vi "RTD Read.vi"(0 "Message Queues":T1, 3 "error in":errorcluster) -> (10 "error out":errorcluster)   [LabVIEW 2018, in "RTD.lvlib"]
uses:
  RTD.lvlib
  support/Message Queue/All Message Queues.ctl
  support/Message Queue/Message Cluster.ctl
  TT Configuration.ctl
  <vilib>/DAQmx/read.llb/DAQmx Read (Analog Wfm 1Chan 1Samp).vi
  <vilib>/DAQmx/create/channels.llb/DAQmx Create Channel (AI-Temperature-RTD).vi
  <vilib>/DAQmx/miscellaneous.llb/DAQmx Fill In Error Info.vi
  support/Message Queue/Enqueue Message (Array).vi
  support/Message Queue/Message Queue.lvlib
  Measure Instrument/Feed Module Engine.lvlib
panel:
  in  "TT Configuration":T2={"physical channels"="cDAQ2Mod4/ai0", "name to assign"="Temp1", "units"=10143} {"units" items=["Deg C"=10143, "Deg F"=10144, "Kelvins"=10325, "Deg R"=10145, "From Custom Scale"=10065]}
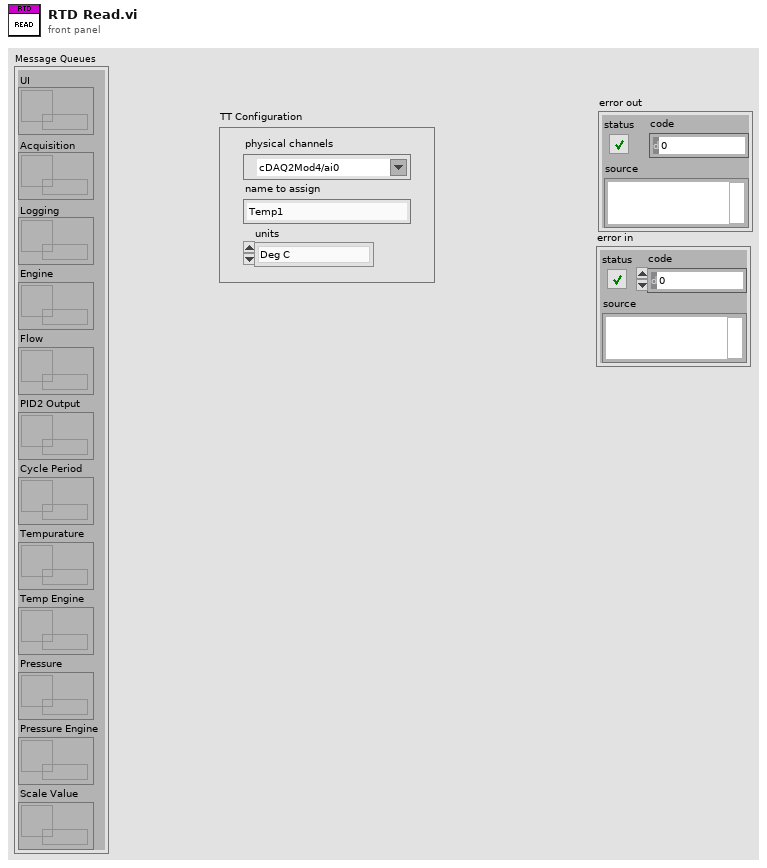
[diagram p1: front panel]
types:
  T1 = typedef "Message Queue.lvlib/All Message Queues.ctl" = cluster{"UI":refnum<queue>, "Acquisition":refnum<queue>, "Logging":refnum<queue>, "Engine":refnum<queue>, "Flow":refnum<queue>, "PID2 Output":refnum<queue>, "Cycle Period":refnum<queue>, "Tempurature":refnum<queue>, "Temp Engine":refnum<queue>, "Pressure":refnum<queue>, "Pressure Engine":refnum<queue>, "Scale Value":refnum<queue>}
  T2 = cluster{"physical channels":tag, "name to assign":string, "units":i32}
  T3 = typedef "RTD.lvlib/TT Configuration.ctl" = cluster{"physical channels":tag, "name to assign":string, "units":i32}
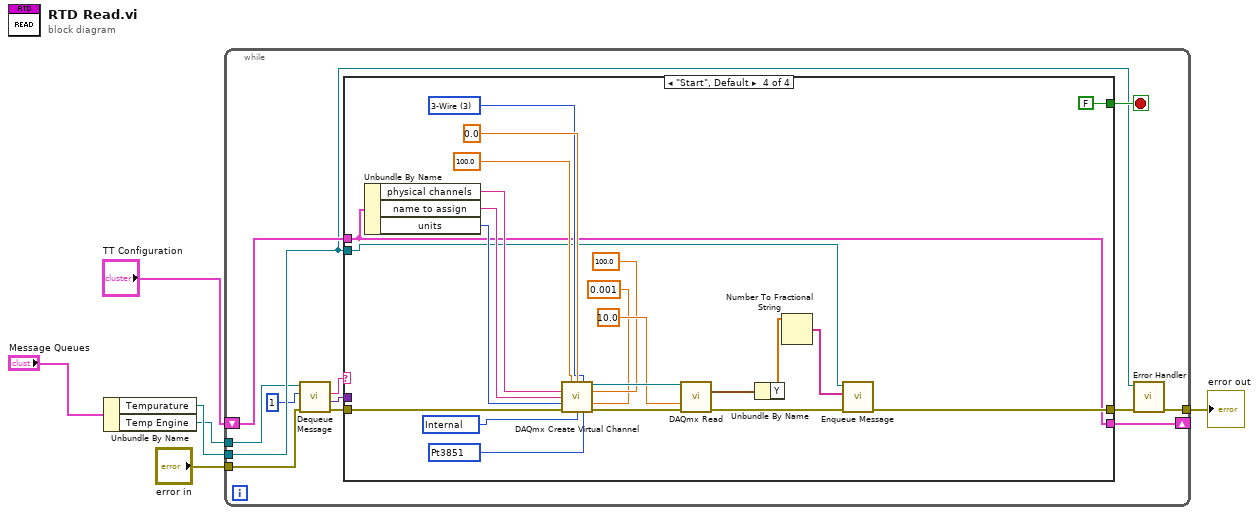
[diagram p0: block diagram]
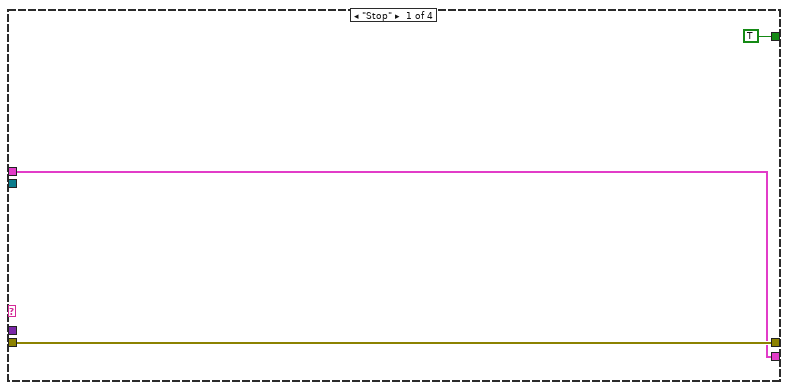
[diagram p2: hidden frame]
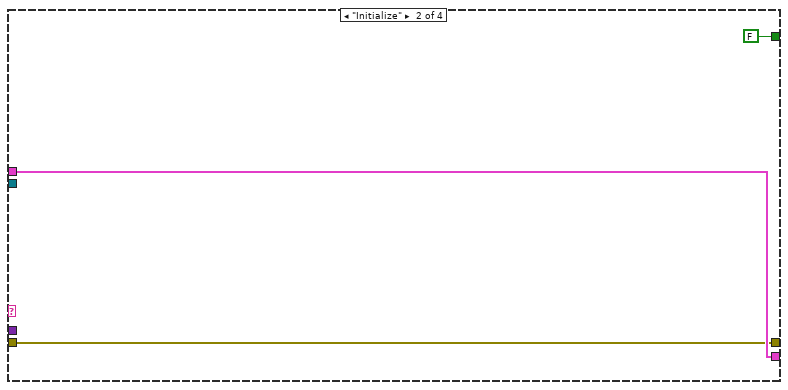
[diagram p3: hidden frame]
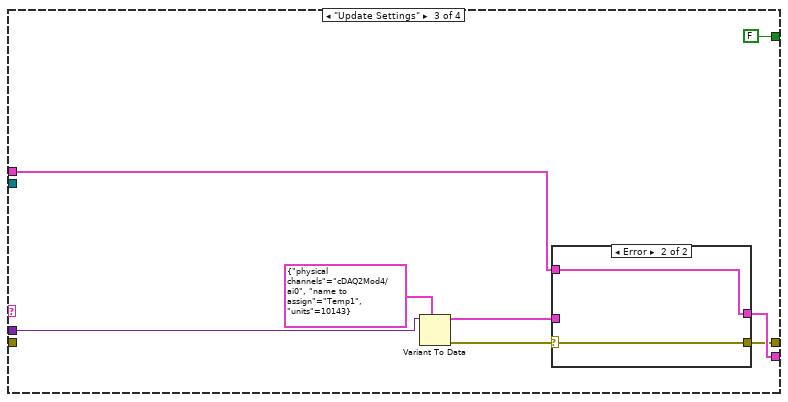
[diagram p4: hidden frame]
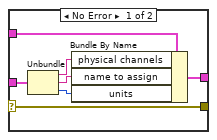
[diagram p5: hidden frame]
diagram:
  n1 = Unbundle By Name("Message Queues") -> ("Tempurature"=w4:refnum<queue>, "Temp Engine"=w1:refnum<queue>)
  n2 = while {
    tunnel: [w8] -> w5
    tunnel: w4 -> [w15]
    shift-right: [w17] -> _
    shift-left: "TT Configuration" -> [w16]
    tunnel: "error in" -> [w14]
    tunnel: w1 -> [w13]
    stop <- w18 stop-if-true
    n3 = call "Dequeue Message.vi"("error in (no error)"=w14, "timeout in ms (-1)"=1, "Message Queue"=w13) -> ("error out"=w12:errorcluster, "Message Data"=w11:variant, "Message"=w10:string)  [unwired: 5 in, 1 out]
    n4 = case shown="\"Start\", Default" w10 {
      tunnel: w12 -> [w21 w23 _ w50]
      tunnel: [w21 w23 w27 w45] -> w9
      tunnel: [TRUE FALSE FALSE FALSE] -> w18
      tunnel: w15 -> [_ _ _ w47]
      tunnel: [w19 w24 w29 w44] -> w17
      tunnel: w16 -> [w19 w24 w28 w44]
      tunnel: w11 -> [_ _ w25 _]
      frame "Stop" {
      }
      frame "Initialize" {
      }
      frame "Update Settings" {
        n5 = Variant To Data(type=T3 {"physical channels"="cDAQ2Mod4/ai0", "name to assign"="Temp1", "units"=10143} ("TT Configuration"), Variant=w25) -> (data=w31:T3, error out=w32:errorcluster)  [unwired: 1 in]
        n6 = case shown="Error" w32 {
          selector: w32 -> [w33 w40]
          tunnel: w28 -> [w39 w41]
          tunnel: w31 -> [w37 _]
          tunnel: [w38 w41] -> w29
          tunnel: [w33 w40] -> w27
          frame No Error {
            n7 = Unbundle(w37) -> ("physical channels"=w36:tag, "name to assign"=w35:string, "units"=w34:i32)
            n8 = Bundle By Name(cluster=w39, "physical channels"=w36, "name to assign"=w35, "units"=w34) -> (w38:T2)
          }
          frame Error {
          }
        }
      }
      frame "Start", Default {
        w55 = 10200 items=["Internal"=10200, "External"=10167, "None"=10230] ("current excitation source")
        w54 = 10071 items=["Pt3750"=12481, "Pt3851"=10071, "Pt3911"=12482, "Pt3916"=10069, "Pt3920"=10053, "Pt3928"=12483, "Custom"=10137] ("rtd type")
        w58 = 3 items=["2-Wire"=2, "3-Wire"=3, "4-Wire"=4] ("resistance configuration")
        n9 = Unbundle By Name(w44) -> ("physical channels"=w53:tag, "name to assign"=w52:string, "units"=w51:i32)
        n10 = call-poly <vilib>:"DAQmx Create Virtual Channel.vi"("maximum value"=100.0, "minimum value"=0.0, "resistance configuration"=w58, "physical channels"=w53, "r0"=100.0, "name to assign"=w52, "units"=w51, "current excitation value"=0.001, "error in"=w50, "current excitation source"=w55, "rtd type"=w54) -> ("task out"=w62:refnum<k21>, "error out"=w63:errorcluster)  [unwired: 3 in]
        n11 = call-poly <vilib>:"DAQmx Read.vi"("task/channels in"=w62, "timeout"=10.0, "error in"=w63) -> ("data"=w49:waveform(dbl), "error out"=w46:errorcluster)  [unwired: 10 in, 1 out]
        n12 = Unbundle By Name(w49) -> ("Y"=w43:dbl[])
        n13 = Number To Fractional String(number=w43) -> (F-format string=w42:string[])  [unwired: 3 in]
        n14 = call-poly "Enqueue Message.vi"("error in (no error)"=w46, "Message Array"=w42, "Message Queue"=w47) -> ("error out"=w45:errorcluster)  [unwired: 7 in, 1 out]
      }
    }
    n15 = call "Error Handler.vi"("error in (no error)"=w9, "Message Queue"=w15) -> ("dup error in"=w8:errorcluster)  [unwired: 8 in, 1 out]
  }
  "error out" <- w5
